vi "Update REF Parameter.vi"(6 "Parameter":T1, 8 "error in":errorcluster, 9 "Value":variant, 10 "Channel":i32, 11 "Instrument.Lockin":refnum<class "Instrument.Lockin.lvclass">) -> (0 "error out":errorcluster, 3 "Instrument.Lockin out":refnum<class "Instrument.Lockin.lvclass">)   [LabVIEW 2019, in "Instrument.Lockin.lvclass"]
uses:
  Instrument.Lockin.lvclass
  Typedefs/REF Parameter--Enum.ctl
  Instrument.Lockin.lvclass/Instrument.Lockin.ctl
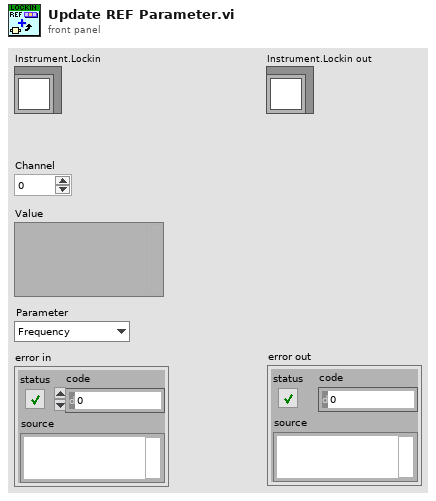
[diagram p1: front panel]
types:
  T1 = typedef "Instrument.Lockin.lvclass/REF Parameter--Enum.ctl" = enum16{"Frequency", "Phase", "Time Constant", "RollOff"}
  T2 = typedef "Instrument.DAQ.lvclass/REF.Channel--Cluster--Array.ctl" = T3[]
  T3 = typedef "Instrument.DAQ.lvclass/REF.Channel--Cluster.ctl" = cluster{"Enable?":bool, "Channel":i32, "Frequency":dbl, "Phase":dbl, "TC":dbl, "Roll-Off":i32}
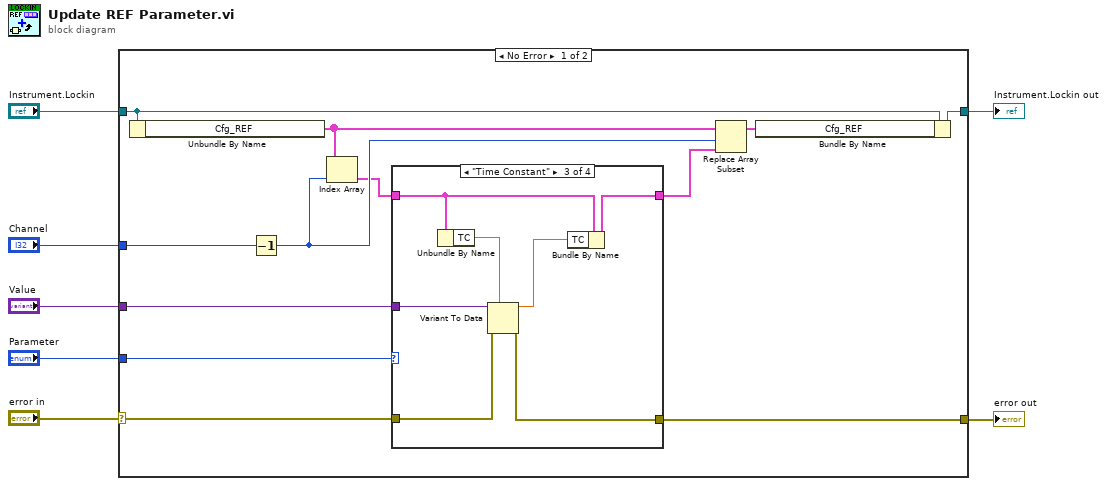
[diagram p0: block diagram]
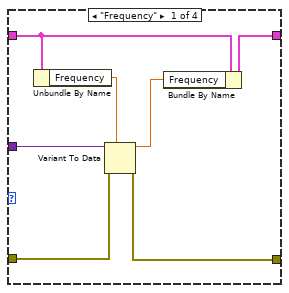
[diagram p2: hidden frame]
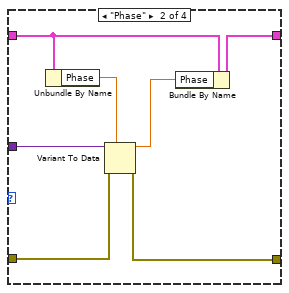
[diagram p3: hidden frame]
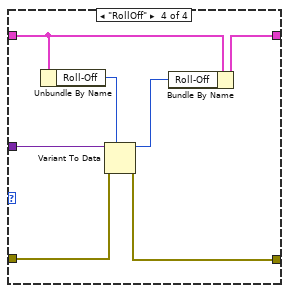
[diagram p4: hidden frame]
diagram:
  n1 = case shown="No Error" "error in" {
    selector: "error in" -> [w11 w49]
    tunnel: "Channel" -> [w19 _]
    tunnel: "Value" -> [w18 _]
    tunnel: [w17 w49] -> w5
    tunnel: "Parameter" -> [w16 _]
    tunnel: "Instrument.Lockin" -> [w13 w48]
    tunnel: [w12 w48] -> w2
    frame No Error {
      n2 = Unbundle By Name(w13) -> ("Cfg_REF"=w14:T2)
      n3 = Decrement(x=w19) -> (x-1=w15:i32)
      n4 = Index Array(array=w14, index=w15) -> (element=w8:T3)
      n5 = case shown="\"Time Constant\"" w16 {
        tunnel: w8 -> [w26 w33 w40 w47]
        tunnel: w11 -> [w21 w28 w35 w42]
        tunnel: w18 -> [w23 w30 w37 w44]
        tunnel: [w20 w27 w34 w41] -> w17
        tunnel: [w22 w29 w36 w43] -> w9
        frame "Frequency" {
          n6 = Unbundle By Name(w26) -> ("Frequency"=w25:dbl)
          n7 = Variant To Data(error in=w21, type=w25, Variant=w23) -> (data=w24:dbl, error out=w20:errorcluster)
          n8 = Bundle By Name(cluster=w26, "Frequency"=w24) -> (w22:T3)
        }
        frame "Phase" {
          n9 = Unbundle By Name(w33) -> ("Phase"=w32:dbl)
          n10 = Variant To Data(error in=w28, type=w32, Variant=w30) -> (data=w31:dbl, error out=w27:errorcluster)
          n11 = Bundle By Name(cluster=w33, "Phase"=w31) -> (w29:T3)
        }
        frame "Time Constant" {
          n12 = Unbundle By Name(w40) -> ("TC"=w39:dbl)
          n13 = Variant To Data(error in=w35, type=w39, Variant=w37) -> (data=w38:dbl, error out=w34:errorcluster)
          n14 = Bundle By Name(cluster=w40, "TC"=w38) -> (w36:T3)
        }
        frame "RollOff" {
          n15 = Unbundle By Name(w47) -> ("Roll-Off"=w46:i32)
          n16 = Variant To Data(error in=w42, type=w46, Variant=w44) -> (data=w45:i32, error out=w41:errorcluster)
          n17 = Bundle By Name(cluster=w47, "Roll-Off"=w45) -> (w43:T3)
        }
      }
      n18 = Replace Array Subset(array=w14, new element=w9, index=w15) -> (w10:T2)
      n19 = Bundle By Name(cluster=w13, "Cfg_REF"=w10) -> (w12:refnum<class "Instrument.Lockin.lvclass">)
    }
    frame Error {
    }
  }
  "Instrument.Lockin out" <- w2
  "error out" <- w5
